vi "beam cup control.vi"() -> ()   [LabVIEW 2016, in "Top Level.lvlib"]
doc: "This vi is used to control the cups and apertures in the ams beamline."
uses:
  Top Level.lvlib
  controls/FC beamlines.ctl
  sub-VIs/sub-VIs.lvlib
  controls/beamline sections.lvlib
panel:
  in  "Which Beamline?":T1
  out "R45 detector cup":string="OUT"
  out "R45 detector aperture":string="IN"
  out "R45 switch image cup":string="IN"
  out "R45 switch aperture":string="OUT"
  in  "R30 detector ap":bool=TRUE
  out "R30 detector aperture":string="IN"
  out "R30 Detector cup rd":string="OUT"
  out "R30 switch aperture":string="IN"
  in  "R30 Image ap":bool=TRUE
  out "R30 switch image cup":string="OUT"
  out "analyze image cup rd":string="OUT"
  out "tank exit cup  rd":string="OUT"
  out "tank entrance cup  rd":string="OUT"
  out "low energy cup":string="OUT"
  out "injector image aperture":string="IN"
  out "injector cup":string="OUT"
  in  "r45 det cup":bool
  in  "R45  det ap":bool
  in  "r45 switch image cup":bool=TRUE
  in  "R45 #1 ap":bool
  out "Terminal Voltage":dbl=8.333384070396422 format="%#_4g"
  in  "R30 det cup":bool
  in  "Switch magnet cup":bool
  in  "Analyze image cup":bool
  in  "Tank exit cup":bool
  in  "Tank Entrance cup":bool
  in  "Low end waist  cup":bool=TRUE
  in  "Low end waist ap":bool
  in  "INJ Image ap":bool
  in  "Inj Image cup":bool
  out "date/time string":string="3/16/2012  11:07 AM"
  out "Error out":errorcluster
  in  "stop":bool
  # "Faraday cup Controls"
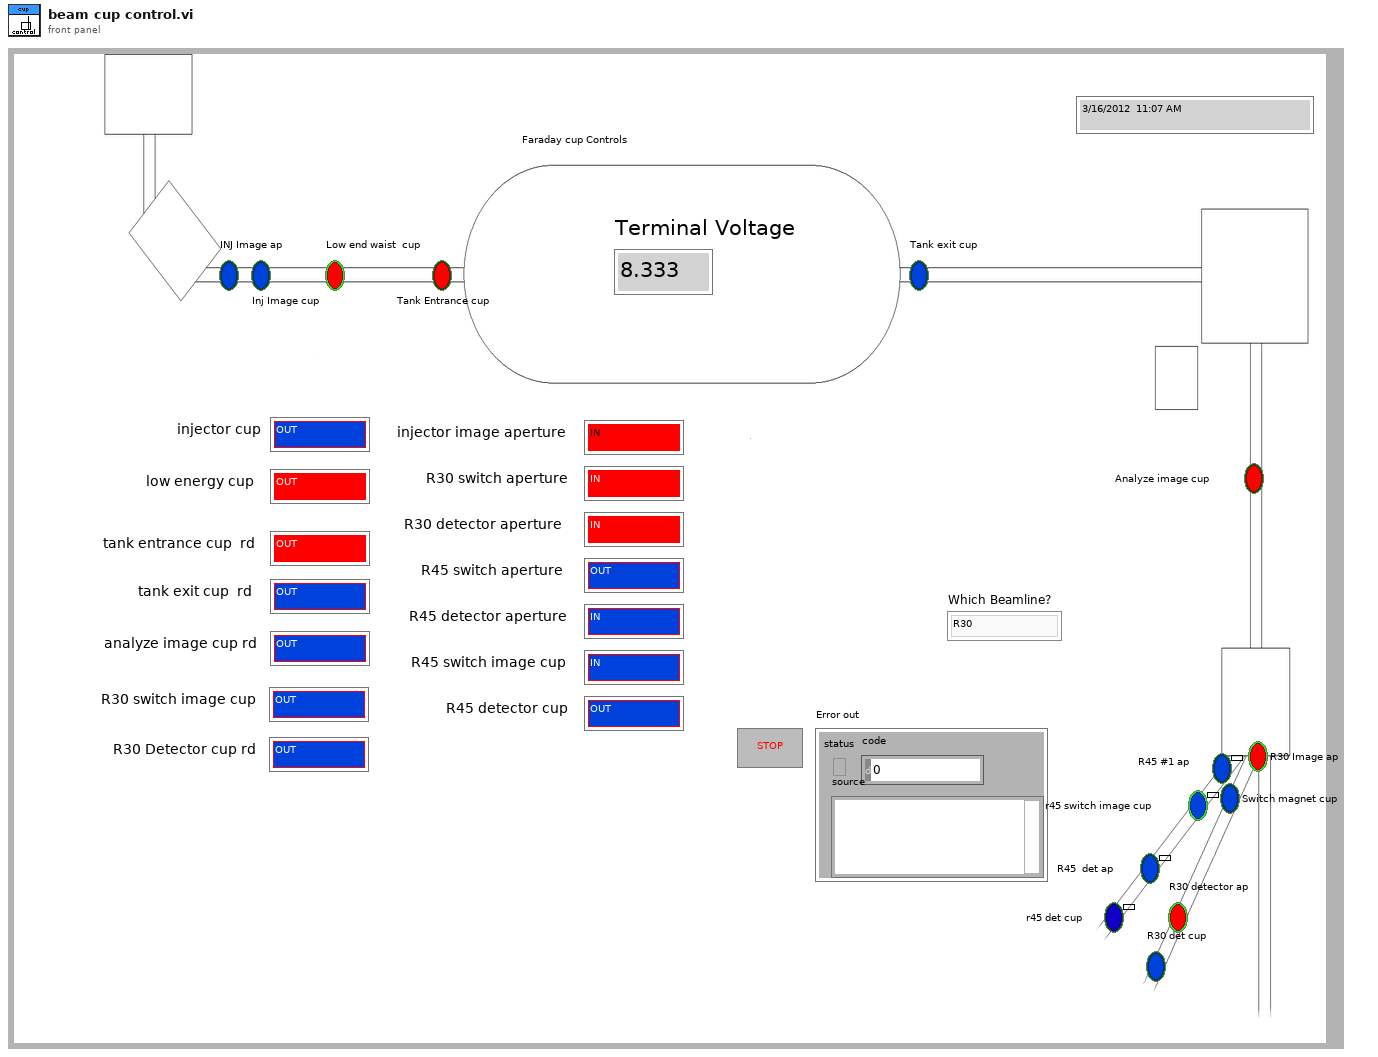
[diagram p1: front panel]
types:
  T1 = typedef "FC beamlines.ctl" = enum16{"R30", "R45"}
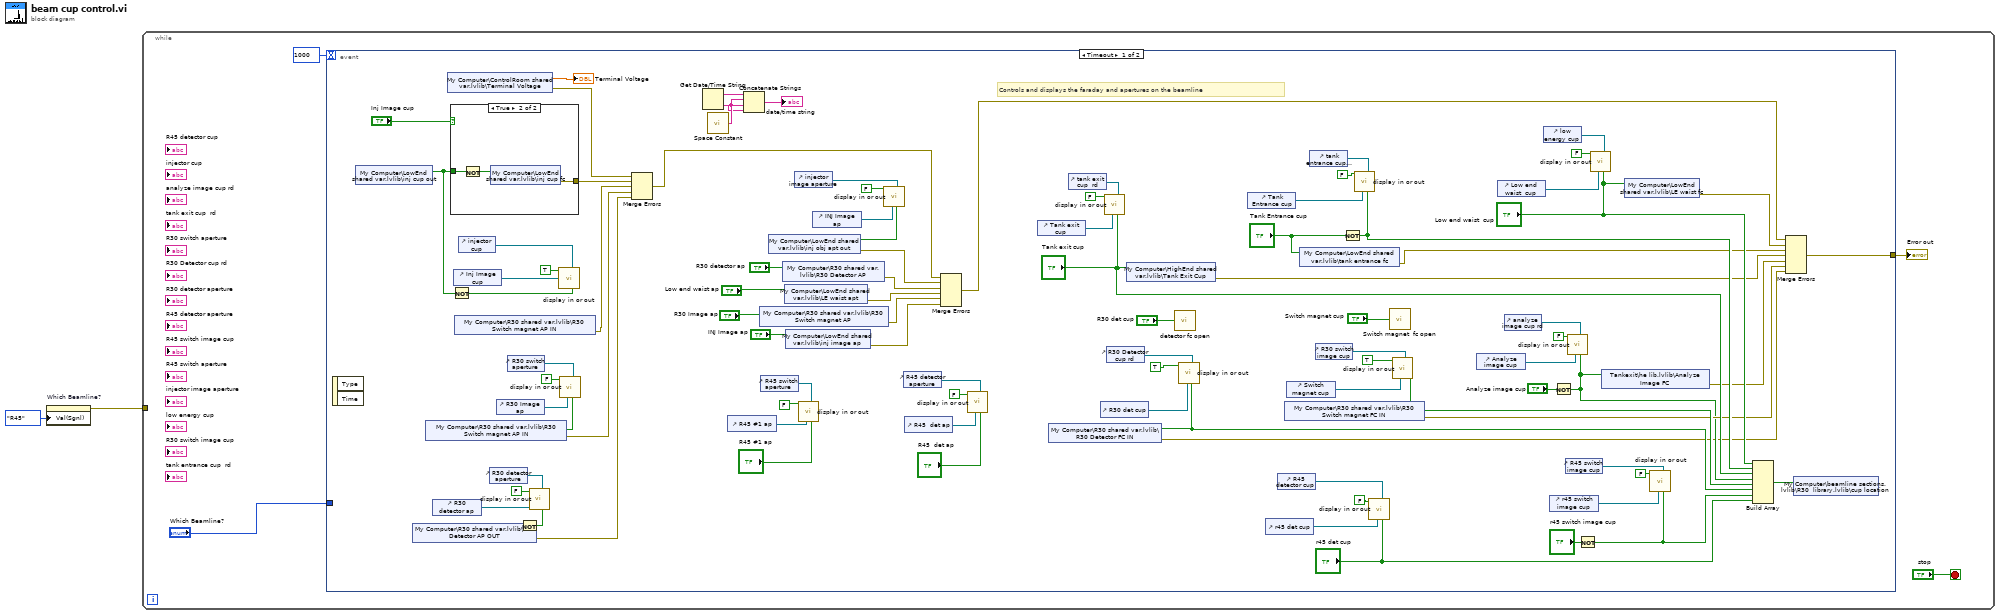
[diagram p0: block diagram]
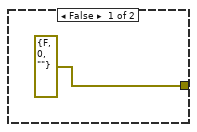
[diagram p2: hidden frame]
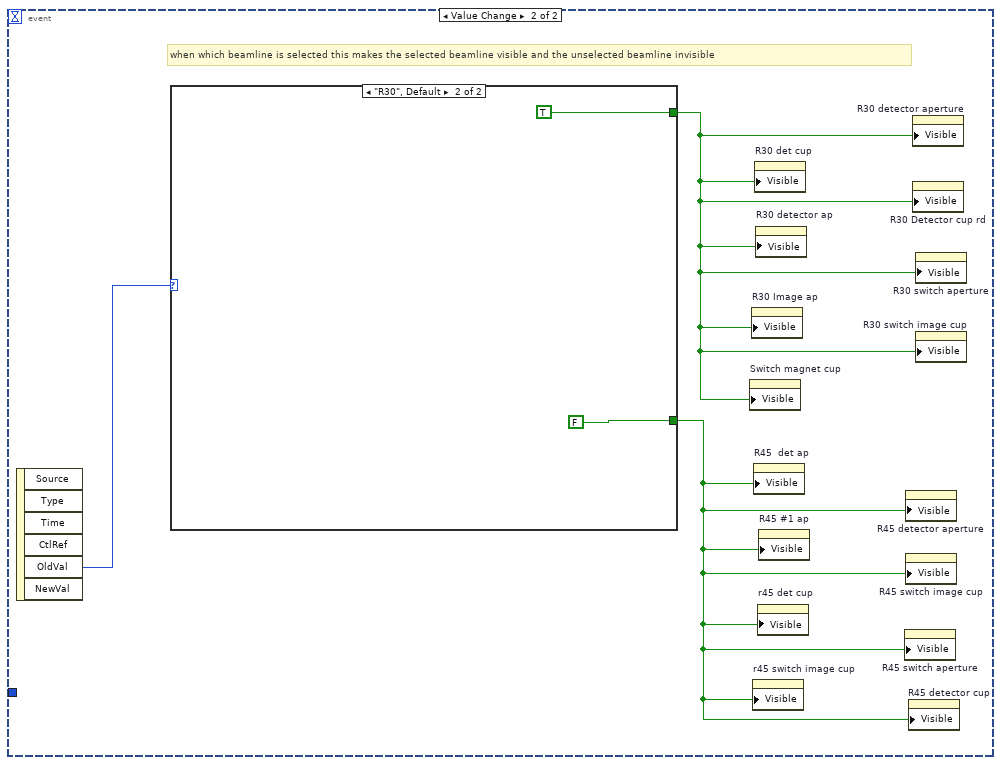
[diagram p3: hidden frame]
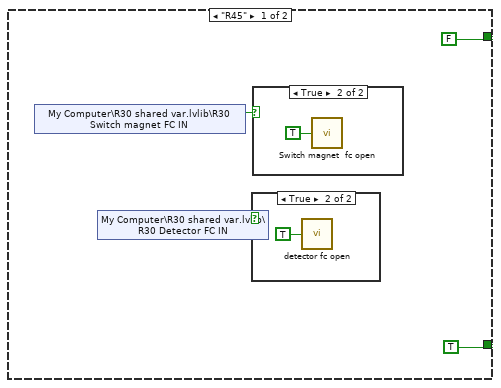
[diagram p4: hidden frame]
diagram:
  n1 = property on="Which Beamline?" class="Enum (strict)"("Val(Sgnl)"=FC_beamlines."R45" ("Value (Signaling)")) -> (error out=w2:errorcluster)  [unwired: 2 in, 1 out]
  n2 = while {
    tunnel: w2 -> [_]
    stop <- "stop" stop-if-true
    n3 = event shown="[0] Timeout" {
      selector: _ -> [_ _]
      dyn-events: _ -> [_ _]
      timeout: 1000 -> [_ _]
      tunnel: [w14 _] -> w4
      tunnel: "Which Beamline?" -> [_ _]
      event Timeout {
        # "Controls and displays the faraday and apertures on the beamline"
        n4 = event-data() -> ()  [unwired: 1 in, 2 out]
        n5 = shared-variable "My Computer\\LowEnd shared var.lvlib\\inj cup out"() -> (w26:bool)  [unwired: 1 in, 1 out]
        n6 = shared-variable "My Computer\\R30 shared var.lvlib\\R30 Detector AP OUT"() -> (w60:bool, error out=w18:errorcluster)  [unwired: 1 in]
        n7 = shared-variable "My Computer\\R30 shared var.lvlib\\R30 Switch magnet AP IN"() -> (w61:bool, error out=w19:errorcluster)  [unwired: 1 in]
        n8 = control-ref of="R30 detector ap"() -> (w63:refnum<vi>)
        n9 = shared-variable "My Computer\\ControlRoom shared var.lvlib\\Terminal Voltage"() -> (→"Terminal Voltage":dbl, error out=w25:errorcluster)  [unwired: 1 in]
        n10 = case shown="True" "Inj Image cup" {
          tunnel: [errorcluster {"status"=FALSE, "code"=0, "source"=""} ("error IO") w103] -> w24
          tunnel: w26 -> [_ w102]
          frame False {
          }
          frame True {
            n11 = Not(x=w102) -> (.not. x?=w101:bool)
            n12 = shared-variable "My Computer\\LowEnd shared var.lvlib\\inj cup fc"(w101) -> (error out=w103:errorcluster)  [unwired: 1 in]
          }
        }
        n13 = Not(x=w26) -> (.not. x?=w27:bool)
        n14 = control-ref of="Inj Image cup"() -> (w94:refnum<vi>)
        n15 = shared-variable "My Computer\\R30 shared var.lvlib\\R30 Switch magnet AP IN"() -> (error out=w23:errorcluster)  [unwired: 1 in, 1 out]
        n16 = control-ref of="injector cup"() -> (w95:refnum<vi>)
        n17 = control-ref of="R30 detector aperture"() -> (w62:refnum<vi>)
        n18 = control-ref of="R30 Image ap"() -> (w70:refnum<vi>)
        n19 = control-ref of="R30 switch aperture"() -> (w71:refnum<vi>)
        n20 = Not(x=w60) -> (.not. x?=w59:bool)
        n21 = call "display in or out.vi"("device in beam?"=w59, "in or out display Refnum"=w62, "device control Refnum"=w63, "use color control"=FALSE) -> ()  [unwired: 7 in, 1 out]
        n22 = call "display in or out.vi"("device in beam?"=w27, "in or out display Refnum"=w95, "device control Refnum"=w94, "use color control"=TRUE) -> ()  [unwired: 7 in, 1 out]
        n23 = call "display in or out.vi"("device in beam?"=w61, "in or out display Refnum"=w71, "device control Refnum"=w70, "use color control"=FALSE) -> ()  [unwired: 7 in, 1 out]
        n24 = Merge Errors(w25, w24, w23, w19, w18) -> (w17:errorcluster)
        n25 = Get Date/Time String() -> (date string=w99:string, time string=w96:string)  [unwired: 3 in]
        n26 = call <vilib>:"Space Constant.vi"() -> ("String"=w97:string)
        n27 = control-ref of="R45 #1 ap"() -> (w57:refnum<vi>)
        n28 = Concatenate Strings(w99, w97, w97, w96) -> (→"date/time string":string)
        n29 = shared-variable "My Computer\\R30 shared var.lvlib\\R30 Switch magnet AP"("R30 Image ap") -> (error out=w22:errorcluster)  [unwired: 1 in]
        n30 = control-ref of="R45 switch aperture"() -> (w56:refnum<vi>)
        n31 = shared-variable "My Computer\\LowEnd shared var.lvlib\\inj obj apt out"() -> (w29:bool, error out=w21:errorcluster)  [unwired: 1 in]
        n32 = shared-variable "My Computer\\R30 shared var.lvlib\\R30 Detector AP"("R30 detector ap") -> (error out=w40:errorcluster)  [unwired: 1 in]
        n33 = shared-variable "My Computer\\LowEnd shared var.lvlib\\LE waist apt"("Low end waist ap") -> (error out=w39:errorcluster)  [unwired: 1 in]
        n34 = shared-variable "My Computer\\LowEnd shared var.lvlib\\inj image ap"("INJ Image ap") -> (error out=w20:errorcluster)  [unwired: 1 in]
        n35 = control-ref of="injector image aperture"() -> (w93:refnum<vi>)
        n36 = call "display in or out.vi"("device in beam?"="R45 #1 ap", "in or out display Refnum"=w56, "device control Refnum"=w57, "use color control"=FALSE) -> ()  [unwired: 7 in, 1 out]
        n37 = control-ref of="INJ Image ap"() -> (w92:refnum<vi>)
        n38 = call "display in or out.vi"("device in beam?"=w29, "in or out display Refnum"=w93, "device control Refnum"=w92, "use color control"=FALSE) -> ()  [unwired: 7 in, 1 out]
        n39 = control-ref of="R45 detector aperture"() -> (w51:refnum<vi>)
        n40 = control-ref of="R45  det ap"() -> (w50:refnum<vi>)
        n41 = Merge Errors(w17, w21, w40, w39, w22, w20) -> (w15:errorcluster)
        n42 = call "display in or out.vi"("device in beam?"="R45  det ap", "in or out display Refnum"=w51, "device control Refnum"=w50, "use color control"=FALSE) -> ()  [unwired: 7 in, 1 out]
        n43 = control-ref of="Tank exit cup"() -> (w81:refnum<vi>)
        n44 = shared-variable "My Computer\\R30 shared var.lvlib\\R30 Detector FC IN"() -> (w65:bool, error out=w7:errorcluster)  [unwired: 1 in]
        n45 = control-ref of="tank exit cup  rd"() -> (w80:refnum<vi>)
        n46 = control-ref of="R30 det cup"() -> (w67:refnum<vi>)
        n47 = call "display in or out.vi"("device in beam?"="Tank exit cup", "in or out display Refnum"=w80, "device control Refnum"=w81, "use color control"=FALSE) -> ()  [unwired: 7 in, 1 out]
        n48 = control-ref of="R30 Detector cup rd"() -> (w68:refnum<vi>)
        n49 = shared-variable "My Computer\\HighEnd shared var.lvlib\\Tank Exit Cup"("Tank exit cup") -> (error out=w11:errorcluster)  [unwired: 1 in]
        n50 = call "detector fc open.vi"("Faraday cup"="R30 det cup") -> ()
        n51 = call "display in or out.vi"("device in beam?"=w65, "in or out display Refnum"=w68, "device control Refnum"=w67, "use color control"=TRUE) -> ()  [unwired: 7 in, 1 out]
        n52 = control-ref of="Tank Entrance cup"() -> (w85:refnum<vi>)
        n53 = control-ref of="r45 det cup"() -> (w46:refnum<vi>)
        n54 = control-ref of="R45 detector cup"() -> (w45:refnum<vi>)
        n55 = shared-variable "My Computer\\R30 shared var.lvlib\\R30 Switch magnet FC IN"() -> (w72:bool, error out=w9:errorcluster)  [unwired: 1 in]
        n56 = control-ref of="Switch magnet cup"() -> (w74:refnum<vi>)
        n57 = shared-variable "My Computer\\LowEnd shared var.lvlib\\tank entrance fc"("Tank Entrance cup") -> (error out=w12:errorcluster)  [unwired: 1 in]
        n58 = control-ref of="tank entrance cup  rd"() -> (w86:refnum<vi>)
        n59 = control-ref of="R30 switch image cup"() -> (w73:refnum<vi>)
        n60 = Not(x="Tank Entrance cup") -> (.not. x?=w41:bool)
        n61 = call "display in or out.vi"("device in beam?"=w41, "in or out display Refnum"=w86, "device control Refnum"=w85, "use color control"=FALSE) -> ()  [unwired: 7 in, 1 out]
        n62 = call "display in or out.vi"("device in beam?"="r45 det cup", "in or out display Refnum"=w45, "device control Refnum"=w46, "use color control"=FALSE) -> ()  [unwired: 7 in, 1 out]
        n63 = call "Switch magnet  fc open.vi"("Faraday cup"="Switch magnet cup") -> ()
        n64 = call "display in or out.vi"("device in beam?"=w72, "in or out display Refnum"=w73, "device control Refnum"=w74, "use color control"=TRUE) -> ()  [unwired: 7 in, 1 out]
        n65 = control-ref of="Analyze image cup"() -> (w77:refnum<vi>)
        n66 = control-ref of="Low end waist  cup"() -> (w88:refnum<vi>)
        n67 = control-ref of="analyze image cup rd"() -> (w78:refnum<vi>)
        n68 = control-ref of="low energy cup"() -> (w87:refnum<vi>)
        n69 = control-ref of="r45 switch image cup"() -> (w53:refnum<vi>)
        n70 = Not(x="Analyze image cup") -> (.not. x?=w8:bool)
        n71 = control-ref of="R45 switch image cup"() -> (w54:refnum<vi>)
        n72 = call "display in or out.vi"("device in beam?"=w8, "in or out display Refnum"=w78, "device control Refnum"=w77, "use color control"=FALSE) -> ()  [unwired: 7 in, 1 out]
        n73 = Not(x="r45 switch image cup") -> (.not. x?=w30:bool)
        n74 = call "display in or out.vi"("device in beam?"="Low end waist  cup", "in or out display Refnum"=w87, "device control Refnum"=w88, "use color control"=FALSE) -> ()  [unwired: 7 in, 1 out]
        n75 = shared-variable "Tankexit\\he lib.lvlib\\Analyze Image FC"(w8) -> (error out=w10:errorcluster)  [unwired: 1 in]
        n76 = shared-variable "My Computer\\LowEnd shared var.lvlib\\LE waist fc"("Low end waist  cup") -> (error out=w13:errorcluster)  [unwired: 1 in]
        n77 = call "display in or out.vi"("device in beam?"=w30, "in or out display Refnum"=w54, "device control Refnum"=w53, "use color control"=FALSE) -> ()  [unwired: 7 in, 1 out]
        n78 = Build Array("Low end waist  cup", w41, "Tank exit cup", w8, w72, w65, w30, "r45 det cup") -> (w31:bool[])
        n79 = Merge Errors(w15, w13, w12, w11, w10, w9, w7) -> (w14:errorcluster)
        n80 = shared-variable "My Computer\\beamline sections.lvlib\\R30  library.lvlib\\cup location"(w31) -> ()  [unwired: 1 in, 1 out]
      }
      event Value Change {
        # "when which beamline is selected this makes the selected beamline visible and the unselected beamline invisible"
        n81 = event-data() -> ("OldVal"=w106:T1)  [unwired: 1 in, 5 out]
        n82 = case shown="\"R30\", Default" w106 {
          tunnel: [TRUE ("Visible") FALSE ("Visible")] -> w104
          tunnel: [FALSE ("Visible") TRUE ("Visible")] -> w105
          frame "R45" {
            n83 = shared-variable "My Computer\\R30 shared var.lvlib\\R30 Switch magnet FC IN"() -> (w108:bool)  [unwired: 1 in, 1 out]
            n84 = shared-variable "My Computer\\R30 shared var.lvlib\\R30 Detector FC IN"() -> (w107:bool)  [unwired: 1 in, 1 out]
            n85 = case shown="True" w107 {
              frame False {
              }
              frame True {
                n86 = call "detector fc open.vi"("Faraday cup"=TRUE ("inj cup fc")) -> ()
              }
            }
            n87 = case shown="True" w108 {
              frame False {
              }
              frame True {
                n88 = call "Switch magnet  fc open.vi"("Faraday cup"=TRUE ("inj cup fc")) -> ()
              }
            }
          }
          frame "R30", Default {
          }
        }
        n89 = property on="Switch magnet cup" class="Bool"("Visible"=w105) -> ()  [unwired: 2 in, 2 out]
        n90 = property on="R30 Image ap" class="Bool (strict)"("Visible"=w105) -> ()  [unwired: 2 in, 2 out]
        n91 = property on="r45 switch image cup" class="Bool (strict)"("Visible"=w104) -> ()  [unwired: 2 in, 2 out]
        n92 = property on="R45  det ap" class="Bool (strict)"("Visible"=w104) -> ()  [unwired: 2 in, 2 out]
        n93 = property on="R30 det cup" class="Bool"("Visible"=w105) -> ()  [unwired: 2 in, 2 out]
        n94 = property on="R30 detector ap" class="Bool (strict)"("Visible"=w105) -> ()  [unwired: 2 in, 2 out]
        n95 = property on="r45 det cup" class="Bool (strict)"("Visible"=w104) -> ()  [unwired: 2 in, 2 out]
        n96 = property on="R45 #1 ap" class="Bool (strict)"("Visible"=w104) -> ()  [unwired: 2 in, 2 out]
        n97 = property on="R45 switch aperture" class="Str"("Visible"=w104) -> ()  [unwired: 2 in, 2 out]
        n98 = property on="R45 detector aperture" class="Str"("Visible"=w104) -> ()  [unwired: 2 in, 2 out]
        n99 = property on="R45 switch image cup" class="Str"("Visible"=w104) -> ()  [unwired: 2 in, 2 out]
        n100 = property on="R45 detector cup" class="Str"("Visible"=w104) -> ()  [unwired: 2 in, 2 out]
        n101 = property on="R30 detector aperture" class="Str"("Visible"=w105) -> ()  [unwired: 2 in, 2 out]
        n102 = property on="R30 Detector cup rd" class="Str"("Visible"=w105) -> ()  [unwired: 2 in, 2 out]
        n103 = property on="R30 switch aperture" class="Str"("Visible"=w105) -> ()  [unwired: 2 in, 2 out]
        n104 = property on="R30 switch image cup" class="Str"("Visible"=w105) -> ()  [unwired: 2 in, 2 out]
      }
    }
    "Error out" <- w4
  }
